vi "Create Table Config.vi"(8 "error in (no error)":errorcluster) -> (0 "error out":errorcluster)   [LabVIEW 2020, in "Settings.lvlib"]
uses:
  Settings.lvlib
  <vilib>/drjdpowell/SQLite Library/SQL Connection/Open (path).vi
  <vilib>/drjdpowell/SQLite Library/SQL Connection/Open (string).vi
  <vilib>/AdvancedString/Path To Command Line String.vi
  <vilib>/drjdpowell/SQLite Library/SQL Connection/Execute SQL (No results).vi
  <vilib>/drjdpowell/SQLite Library/SQL Connection/Connection.lvclass
  <vilib>/drjdpowell/SQLite Library/SQLite.lvlib
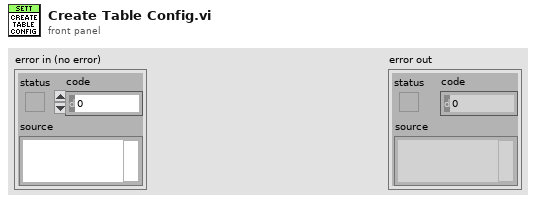
[diagram p1: front panel]
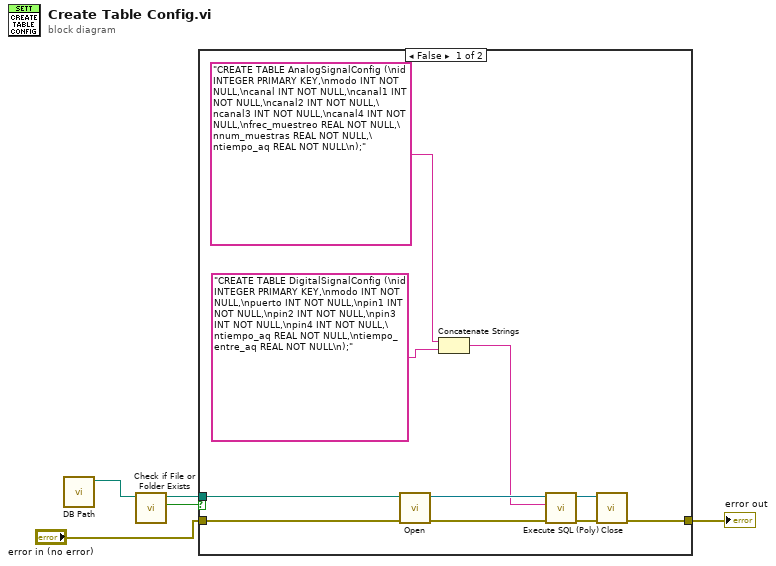
[diagram p0: block diagram]
diagram:
  n1 = call "DB Path.vi"() -> ("appended path"=w1:path)  [unwired: 11 in]
  n2 = call <vilib>:"Check if File or Folder Exists.vi"("path"=w1) -> ("file or folder exists?"=w4:bool, "dup path"=w5:path)  [unwired: 8 in, 1 out]
  n3 = case shown="False" w4 {
    tunnel: w5 -> [w15 _]
    tunnel: "error in (no error)" -> [w10 w16]
    tunnel: [w9 w16] -> w3
    frame False {
      n4 = call-poly <vilib>:"Open.vi"("error in (no error)"=w10, "db file"=w15) -> ("error out"=w14:errorcluster, "SQLite Connection"=w13:refnum<class "Connection.lvclass">)  [unwired: 8 in]
      n5 = Concatenate Strings("CREATE TABLE AnalogSignalConfig (\nid INTEGER PRIMARY KEY,\nmodo INT NOT NULL,\ncanal INT NOT NULL,\ncanal1 INT NOT NULL,\ncanal2 INT NOT NULL,\ncanal3 INT NOT NULL,\ncanal4 INT NOT NULL,\nfrec_muestreo REAL NOT NULL,\nnum_muestras REAL NOT NULL,\ntiempo_aq REAL NOT NULL\n);" ("SQL"), "CREATE TABLE DigitalSignalConfig (\nid INTEGER PRIMARY KEY,\nmodo INT NOT NULL,\npuerto INT NOT NULL,\npin1 INT NOT NULL,\npin2 INT NOT NULL,\npin3 INT NOT NULL,\npin4 INT NOT NULL,\ntiempo_aq REAL NOT NULL,\ntiempo_entre_aq REAL NOT NULL\n);" ("SQL")) -> (w6:string)
      n6 = call-poly <vilib>:"Execute SQL (Poly).vi"("error in (no error)"=w14, "SQL"=w6, "SQLite Connection in"=w13) -> ("error out"=w12:errorcluster, "SQLite Connection"=w11:refnum<class "Connection.lvclass">)  [unwired: 7 in]
      n7 = call-dynamic "Close.vi"("error in (no error)"=w12, "SQLite Connection in"=w11) -> ("error out"=w9:errorcluster)  [unwired: 9 in]
    }
    frame True {
    }
  }
  "error out" <- w3
